vi "Receiver_Example_1.vi"() -> ()   [LabVIEW 2018]
uses:
  <vilib>/picture/picture.llb/imagedata.ctl
panel:
  in  "Numeric":i32
  out "new picture 2":picture
  out "image data 2":T1
  out "BER":dbl
  in  "String":string="PENS"
  out "SNR":dbl
  in  "Modulation parameter":T2
  out "created new?":bool
  out "XY Graph":cdb[](graph)
  out "string 2":string
  out "SIG valid?":bool
  in  "stop":bool
  out "USRP CoercedParamters":T3={"coerced IQ rate"=100000.0, "coerced carrier frequency"=100000.0, "coerced gain"=0.0} {"coerced gain" format="%#_6f"; "coerced carrier frequency" format="%#_6p"; "coerced IQ rate" format="%#_6p"}
  out "error out":errorcluster
  in  "Trigger level":dbl=0.005 format="%f"
  in  "error in (no error)":errorcluster
  in  "USRP ControledParameters":T4={"active antenna"="RX1", "gain"=20.0, "carrier frequency"=915000000.0, "IQ rate"=1000000.0} {"IQ rate" format="%#_6p"; "carrier frequency" format="%#_6p"; "gain" format="%#_6f"}
  in  "device names":refnum<k15>="192.168.10.2"
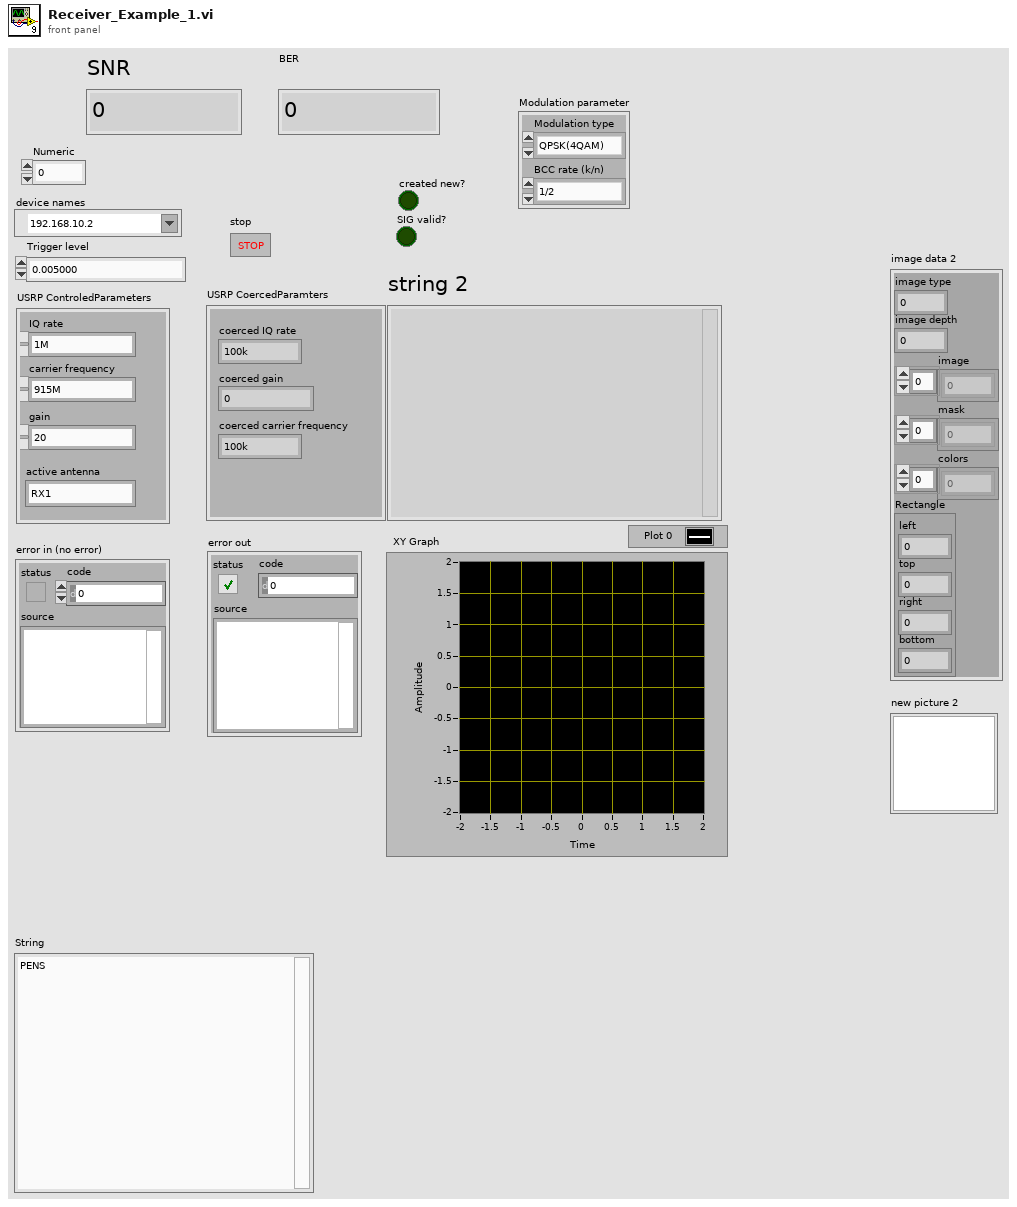
[diagram p1: front panel]
types:
  T1 = typedef "imagedata.ctl" = cluster{"image type":i32, "image depth":i32, "image":u8[], "mask":u8[], "colors":u32[], "Rectangle":cluster{"left":i16, "top":i16, "right":i16, "bottom":i16}}
  T2 = cluster{"Modulation type":enum16{"QPSK(4QAM)", "64QAM", "16QAM", "BPSK"}, "BCC rate (k/n)":enum16{"1/2", "2/3", "3/4"}}
  T3 = cluster{"coerced IQ rate":dbl, "coerced carrier frequency":dbl, "coerced gain":dbl}
  T4 = cluster{"active antenna":string, "gain":dbl, "carrier frequency":dbl, "IQ rate":dbl}
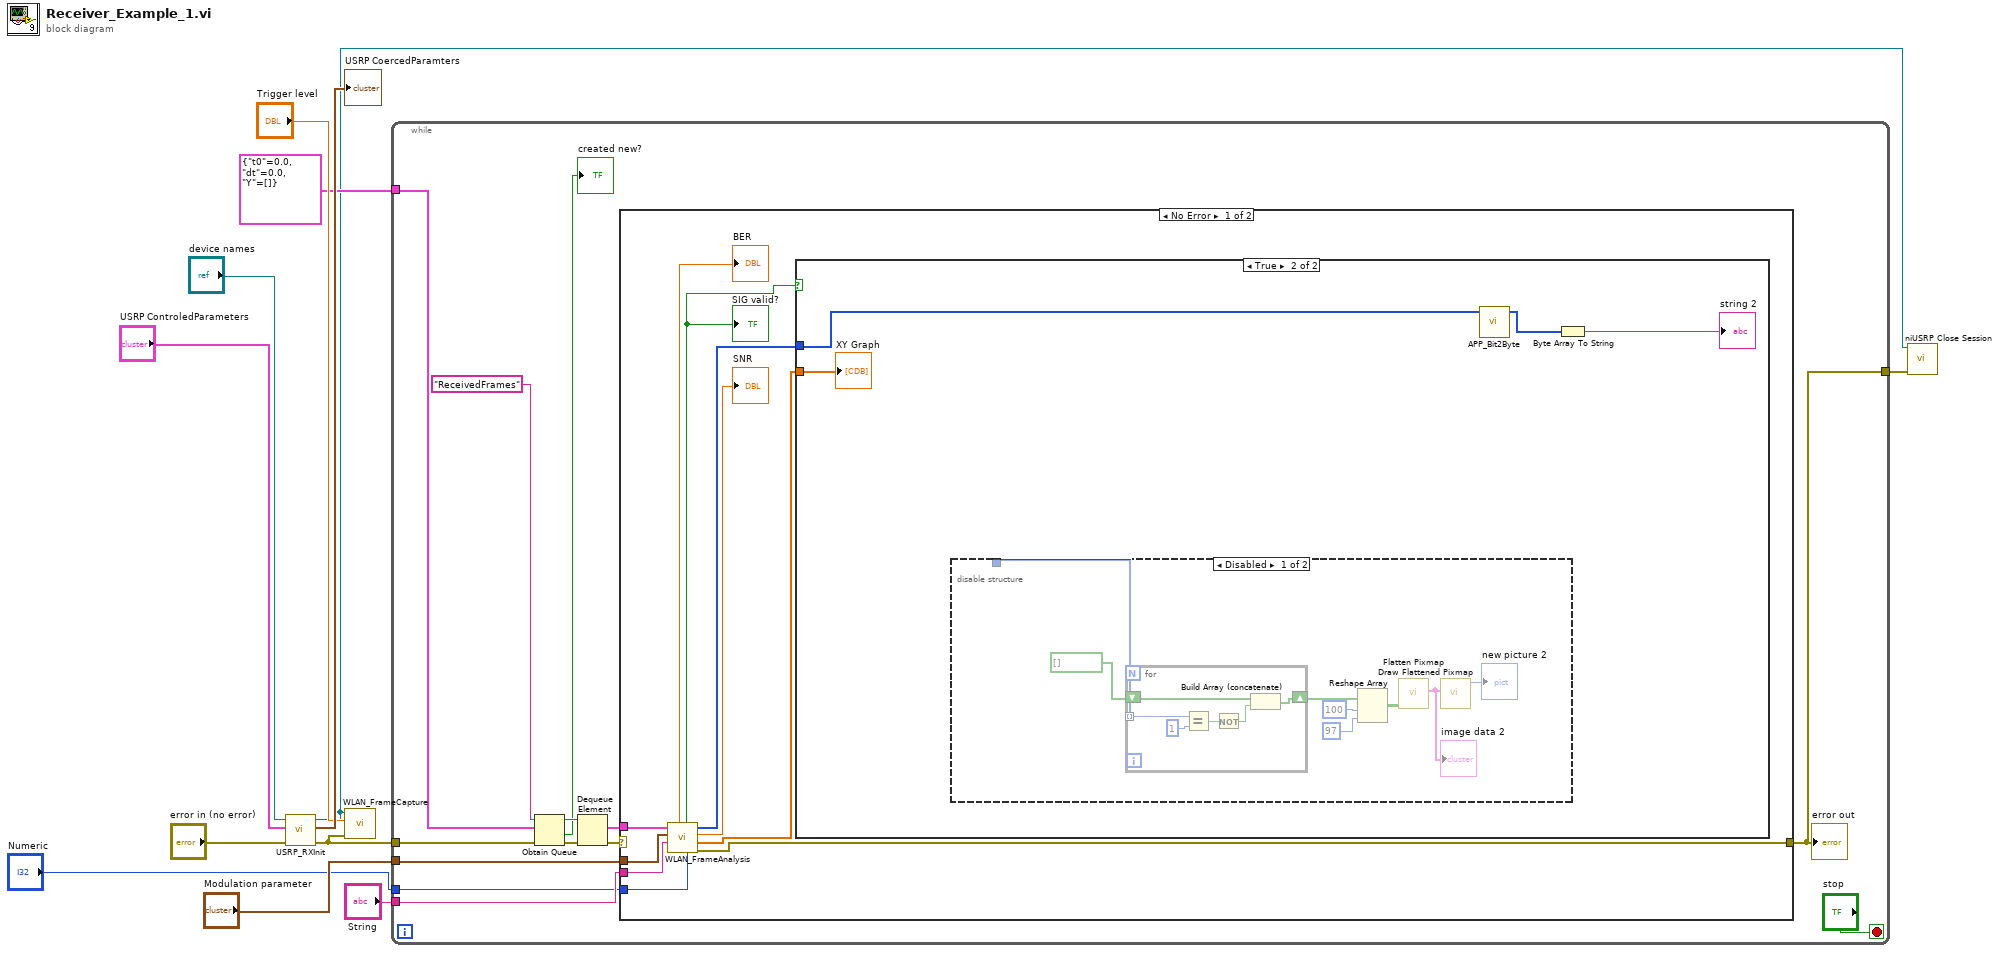
[diagram p0: block diagram]
diagram:
  n1 = call "USRP_RXInit.vi"("device names"="device names", "USRP ControledParameters"="USRP ControledParameters", "error in (no error)"="error in (no error)") -> ("session handle out"=w4:refnum<k15>, "USRP CoercedParamters"=→"USRP CoercedParamters":T3, "error out"=w8:errorcluster)  [unwired: 5 in]
  n2 = call "WLAN_FrameCapture.vi"("error in (no error)"=w8, "Trigger level"="Trigger level", "session handle"=w4) -> ()  [unwired: 8 in]
  n3 = while {
    tunnel: w8 -> [w23]
    tunnel: cluster{"t0":dbl, "dt":dbl, "Y":cdb[]} {"t0"=0.0, "dt"=0.0, "Y"=[]} ("data") -> [w24]
    tunnel: [w16] -> w5
    tunnel: "Modulation parameter" -> [w15]
    tunnel: "String" -> [w14]
    tunnel: "Numeric" -> [w13]
    stop <- "stop" stop-if-true
    n4 = Obtain Queue(name (unnamed)="ReceivedFrames", element data type=w24, error in (no error)=w23) -> (queue out=w22:refnum<queue>, created new?=→"created new?":bool, error out=w19:errorcluster)  [unwired: 2 in]
    n5 = Dequeue Element(queue=w22, error in (no error)=w19) -> (element=w20:cluster{"t0":dbl, "dt":dbl, "Y":cdb[]}, error out=w21:errorcluster)  [unwired: 1 in, 2 out]
    n6 = case shown="No Error" w21 {
      selector: w21 -> [_ w54]
      tunnel: w20 -> [w31 _]
      tunnel: [w32 w54] -> w16
      tunnel: w15 -> [w30 _]
      tunnel: w14 -> [w28 _]
      tunnel: w13 -> [w26 _]
      frame No Error {
        n7 = call "WLAN_FrameAnalysis.vi"("Numeric"=w26, "String"=w28, "Modulation parameter"=w30, "input cluster"=w31) -> ("error out"=w32:errorcluster, "Constellation"=w33:cdb[], "SNR"=→"SNR":dbl, "output bits"=w34:i8[], "SIG valid?"=w35:bool, "BER"=→"BER":dbl)  [unwired: 1 in, 1 out]
        "SIG valid?" <- w35
        n8 = case shown="True" w35 {
          tunnel: w34 -> [_ w38]
          tunnel: w33 -> [_ w39]
          frame False {
          }
          frame True {
            n9 = disable-structure shown="Disabled" {
              disable-tunnel: _ -> [w47 _]
              frame Disabled {
                n10 = for {
                  tunnel: w47 -> [w53] mode=indexing
                  shift-right: [w51] -> w40
                  shift-left: bool[] [] -> [w50]
                  n11 = Equal?(x=w53, y=1) -> (x = y?=w49:bool)
                  n12 = Not(x=w49) -> (.not. x?=w48:bool)
                  n13 = Build Array (concatenate)(w50, w48) -> (w51:bool[])
                }
                n14 = Reshape Array(w40, 100 ("dimension size"), 97 ("dimension size")) -> (w43:bool[][])
                n15 = call <vilib>:"Flatten Pixmap.vi"("1-bit pixmap"=w43) -> ("image data"=w42:T1)  [unwired: 10 in]
                "image data 2" <- w42
                n16 = call <vilib>:"Draw Flattened Pixmap.vi"("image data"=w42) -> ("new picture"=→"new picture 2":picture)  [unwired: 8 in]
              }
              frame Enabled {
              }
            }
            n17 = call "APP_Bit2Byte.vi"("input bit stream"=w38) -> ("output byte stream"=w36:u8[])  [unwired: 9 in, 1 out]
            n18 = Byte Array To String(unsigned byte array=w36) -> (string=→"string 2":string)
            "XY Graph" <- w39
          }
        }
      }
      frame Error {
      }
    }
    "error out" <- w16
  }
  n19 = call <instrlib>:"niUSRP Close Session.vi"("session handle"=w4, "error in (no error)"=w5) -> ()  [unwired: 13 in, 1 out]
